vi "XIPIN_Slice_1_0.vi"   [LabVIEW 2017]
doc: "Slices a number of bits off of Din input. dout = din[from_position : to_position]\n------------------------------------\n<b>Need License</b> : No"
uses:
  <vilib>/rvi/XilinxIP/XIPIN_XNode/niFpgaXIPIN.xnode
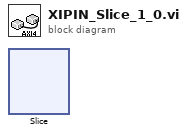
[diagram p0: block diagram]
diagram:
  n1 = xnode ("Slice")() -> ()
